vi "Aadshi.vi"() -> ()   [LabVIEW 2020]
panel:
  out "sorted array":errorcluster[](array[cluster])
  out "size(s) 2":i32
  out "size(s)":i32
  out "Array":i32[](array[numeric])
  out "Numeric":i32
  out "Waveform Graph":dynamicdata(graph)
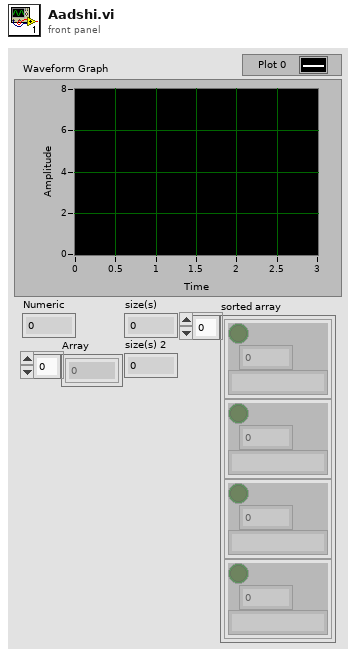
[diagram p1: front panel]
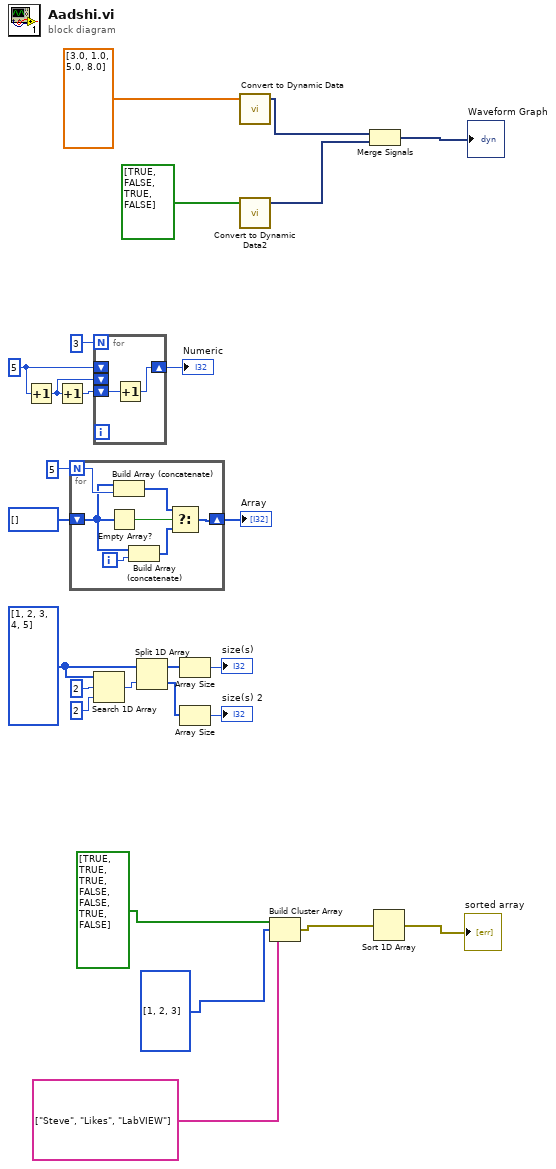
[diagram p0: block diagram]
diagram:
  w11 = i32[] [1, 2, 3, 4, 5]
  w20 = 5
  n1 = Increment(x=w20) -> (x+1=w19:i32)
  n2 = Increment(x=w19) -> (x+1=w18:i32)
  n3 = for {
    N: 5 -> [w32]
    shift-right: [w27] -> w14
    shift-left: i32[] [] -> [w30]
    i -> [w31]
    n4 = Empty Array?(array=w30) -> (empty?=w33:bool)
    n5 = Build Array (concatenate)(w30, w32) -> (w29:i32[])
    n6 = Build Array (concatenate)(w30, w31) -> (w28:i32[])
    n7 = Select(t=w29, s=w33, f=w28) -> (s? t:f=w27:i32[])
  }
  "Array" <- w14
  n8 = for {
    N: 3 -> [_]
    shift-right: [w34] -> w17
    shift-left: w20 -> [_]
    shift-left: w19 -> [_]
    shift-left: w18 -> [w35]
    n9 = Increment(x=w35) -> (x+1=w34:i32)
  }
  "Numeric" <- w17
  n10 = Search 1D Array(1D array=w11, element=2, start index (0)=2) -> (index of element=w8:i32)
  n11 = Split 1D Array(array=w11, index=w8) -> (first subarray=w7:i32[], second subarray=w6:i32[])
  n12 = Array Size(array=w7) -> (size(s)=→"size(s)":i32)
  n13 = Array Size(array=w6) -> (size(s)=→"size(s) 2":i32)
  n14 = call "Convert to Dynamic Data"("Array"=dbl[] [3.0, 1.0, 5.0, 8.0]) -> ("Dynamic Data Type"=w24:dynamicdata)  [unwired: 3 in]
  n15 = call "Convert to Dynamic Data2"("Array"=bool[] [TRUE, FALSE, TRUE, FALSE]) -> ("Dynamic Data Type"=w23:dynamicdata)  [unwired: 3 in]
  n16 = Build Cluster Array(bool[] [TRUE, TRUE, TRUE, FALSE, FALSE, TRUE, FALSE], i32[] [1, 2, 3], string[] ["Steve", "Likes", "LabVIEW"]) -> (w2:errorcluster[])
  n17 = Merge Signals "Merge Signals"(w24, w23) -> (→"Waveform Graph":dynamicdata)
  n18 = Sort 1D Array(array=w2) -> (sorted array=→"sorted array":errorcluster[])
